vi "WMP_ess_CCL.vi"() -> ()   [LabVIEW 2013]
panel:
  out "status":string="就緒"
  out "index":i32
  out "appended path":path=path "C:/Users/TPSOP/Desktop/新增資料夾 (2)/musics/1.mp3"
  in  "Pause Button":bool
  in  "Vol.":i32(slide)=12 min=0 max=100 step=1 scale=0.0..100.0
  in  "Skip Back Button":bool
  in  "Skip Forward Button":bool
  in  "Play Button":bool
  in  "stop":bool
  in  "WindowsMediaPlayer":refnum<k7>(container)
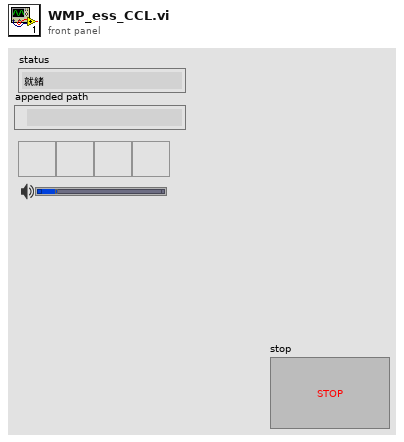
[diagram p1: front panel]
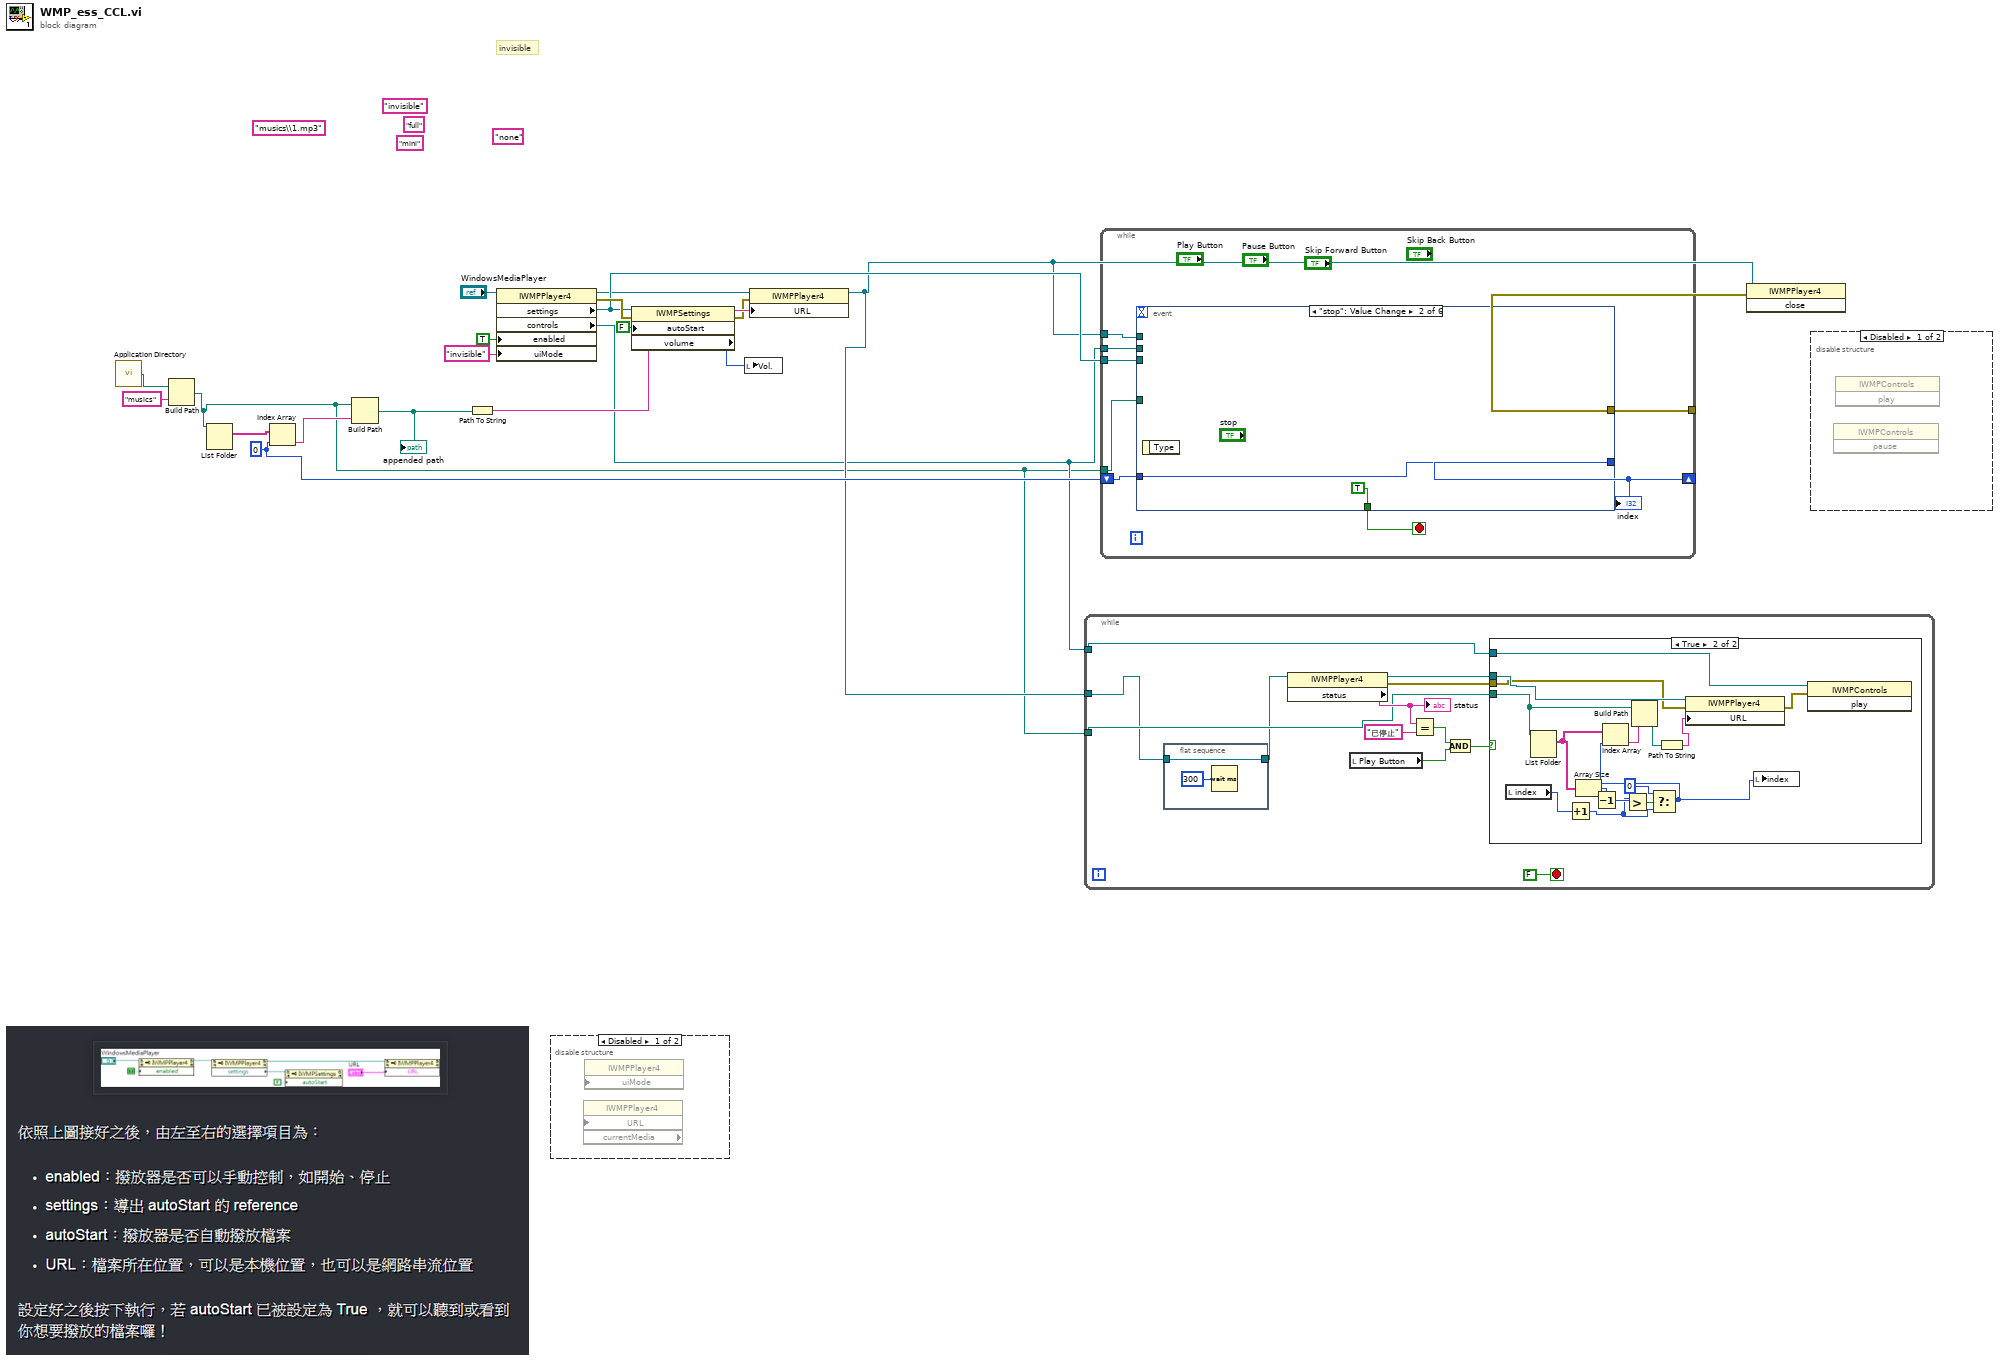
[diagram p0: block diagram]
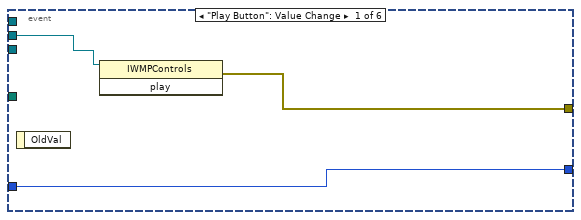
[diagram p5: hidden frame]
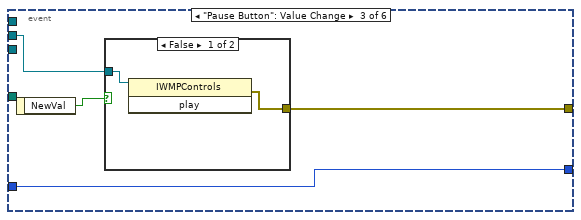
[diagram p6: hidden frame]
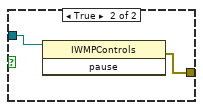
[diagram p7: hidden frame]
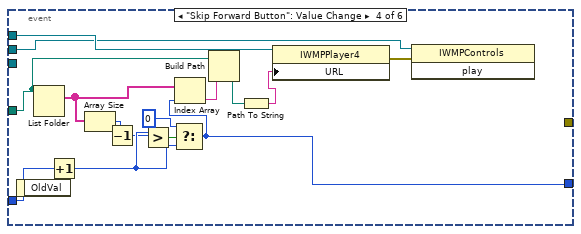
[diagram p8: hidden frame]
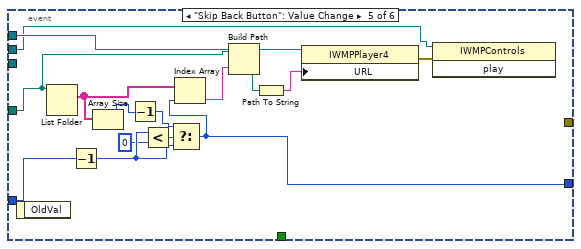
[diagram p9: hidden frame]
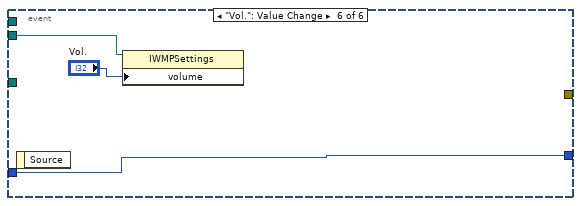
[diagram p10: hidden frame]
diagram:
  (unwired) "invisible" ("uiMode")
  (unwired) "none" ("uiMode")
  (unwired) "mini" ("uiMode")
  (unwired) "full" ("uiMode")
  w5 = 0 ("index")
  (unwired) "musics\\1.mp3" ("name or relative path")
  # "invisible"
  n1 = call <vilib>:"Application Directory.vi"() -> ("Application Directory"=w14:path)
  n2 = Build Path(base path=w14, name or relative path="musics") -> (appended path=w2:path)
  n3 = List Folder(path=w2) -> (filenames=w6:string[])  [unwired: 3 in, 3 out]
  n4 = Index Array(array=w6, index=w5) -> (element=w7:string)
  n5 = Build Path(base path=w2, name or relative path=w7) -> (appended path=w8:path)
  "appended path" <- w8
  n6 = Path To String(path=w8) -> (string=w20:string)
  n7 = property class="IWMPPlayer4"(reference="WindowsMediaPlayer", "enabled"=TRUE, "uiMode"="invisible") -> (reference out=w9:refnum<k7>, error out=w16:errorcluster, "settings"=w12:refnum<k7>, "controls"=w3:refnum<k7>)  [unwired: 1 in]
  n8 = disable-structure shown="Disabled" {
    frame Disabled {
      n9 = property class="IWMPPlayer4" props=["URL", "currentMedia"]() -> ()  [unwired: 3 in, 3 out]
      n10 = property class="IWMPPlayer4" props=["uiMode"]() -> ()  [unwired: 3 in, 2 out]
    }
    frame Enabled {
    }
  }
  n11 = property class="IWMPSettings"(reference=w12, error in=w16, "autoStart"=FALSE) -> (error out=w18:errorcluster, "volume"=w11:i32)  [unwired: 1 out]
  n12 = local write "Vol."(w11) -> ()
  n13 = property class="IWMPPlayer4"(reference=w9, error in=w18, "URL"=w20) -> (reference out=w4:refnum<k7>)  [unwired: 1 out]
  n14 = while {
    tunnel: w4 -> [w22]
    tunnel: w3 -> [w27]
    tunnel: w2 -> [w24]
    stop <- FALSE stop-if-true
    n15 = flat-sequence {
      tunnel: w22 -> [w33]
      tunnel: [w33] -> w21
      frame #0 {
        n16 = Wait (ms)(milliseconds to wait=u32 300 ("millisecond multiple")) -> ()  [unwired: 1 out]
      }
    }
    n17 = property class="IWMPPlayer4"(reference=w21) -> (reference out=w25:refnum<k7>, error out=w23:errorcluster, "status"=w31:string)  [unwired: 1 in]
    "status" <- w31
    n18 = local read "Play Button"() -> (w28:bool)
    n19 = Equal?(x=w31, y="已停止") -> (x = y?=w29:bool)
    n20 = And(x=w29, y=w28) -> (x .and. y?=w26:bool)
    n21 = case shown="True" w26 {
      tunnel: w27 -> [_ w50]
      tunnel: w25 -> [_ w39]
      tunnel: w24 -> [_ w38]
      tunnel: w23 -> [_ w35]
      frame False {
      }
      frame True {
        n22 = local read "index"() -> (w41:i32)
        n23 = List Folder(path=w38) -> (filenames=w42:string[])  [unwired: 3 in, 3 out]
        n24 = Increment(x=w41) -> (x+1=w40:i32)
        n25 = Array Size(array=w42) -> (size(s)=w48:i32)
        n26 = Decrement(x=w48) -> (x-1=w49:i32)
        n27 = Greater?(x=w40, y=w49) -> (0:w43:bool)
        n28 = Select(t=0, s=w43, f=w40) -> (s? t:f=w36:i32)
        n29 = Index Array(array=w42, index=w36) -> (element=w45:string)
        n30 = Build Path(base path=w38, name or relative path=w45) -> (appended path=w46:path)
        n31 = Path To String(path=w46) -> (string=w47:string)
        n32 = property class="IWMPPlayer4"(reference=w39, error in=w35, "URL"=w47) -> (error out=w37:errorcluster)  [unwired: 1 out]
        n33 = local write "index"(w36) -> ()
        n34 = invoke class="IWMPControls" method="play"(reference=w50, error in=w37) -> ()  [unwired: 1 in, 3 out]
      }
    }
  }
  n35 = while {
    tunnel: w3 -> [w58]
    tunnel: [w57] -> w17
    tunnel: w12 -> [w55]
    shift-right: [w51] -> _
    shift-left: w5 -> [w54]
    tunnel: w2 -> [w53]
    tunnel: w4 -> [w52]
    stop <- w56 stop-if-true
    n36 = event shown="[1] \"stop\": Value Change" {
      selector: _ -> [_ _ _ _ _ _]
      dyn-events: _ -> [_ _ _ _ _ _]
      timeout: _ -> [_ _ _ _ _ _]
      tunnel: w58 -> [w61 _ w66 w73 w87 _]
      tunnel: [w60 _ w65 _ _ _] -> w57
      tunnel: [_ TRUE _ _ _ _] -> w56
      tunnel: w55 -> [_ _ _ _ _ w103]
      tunnel: w54 -> [w59 w62 w64 w85 w100 w102]
      tunnel: w53 -> [_ _ _ w79 w93 _]
      tunnel: w52 -> [_ _ _ w86 w101 _]
      tunnel: [w59 w62 w64 w80 w95 w102] -> w51
      event "Play Button": Value Change {
        n37 = event-data() -> ()  [unwired: 1 in, 1 out]
        n38 = invoke class="IWMPControls" method="play"(reference=w61) -> (error out=w60:errorcluster)  [unwired: 2 in, 2 out]
      }
      event "stop": Value Change {
        n39 = event-data() -> ()  [unwired: 1 in, 1 out]
      }
      event "Pause Button": Value Change {
        n40 = event-data() -> ("NewVal"=w67:bool)  [unwired: 1 in]
        n41 = case shown="False" w67 {
          tunnel: w66 -> [w68 w71]
          tunnel: [w69 w70] -> w65
          frame False {
            n42 = invoke class="IWMPControls" method="play"(reference=w68) -> (error out=w69:errorcluster)  [unwired: 2 in, 2 out]
          }
          frame True {
            n43 = invoke class="IWMPControls" method="pause"(reference=w71) -> (error out=w70:errorcluster)  [unwired: 2 in, 2 out]
          }
        }
      }
      event "Skip Forward Button": Value Change {
        n44 = event-data() -> ()  [unwired: 1 in, 1 out]
        n45 = List Folder(path=w79) -> (filenames=w84:string[])  [unwired: 3 in, 3 out]
        n46 = Increment(x=w85) -> (x+1=w82:i32)
        n47 = Array Size(array=w84) -> (size(s)=w75:i32)
        n48 = Decrement(x=w75) -> (x-1=w74:i32)
        n49 = Greater?(x=w82, y=w74) -> (0:w83:bool)
        n50 = Select(t=0, s=w83, f=w82) -> (s? t:f=w80:i32)
        n51 = Index Array(array=w84, index=w80) -> (element=w78:string)
        n52 = Build Path(base path=w79, name or relative path=w78) -> (appended path=w77:path)
        n53 = Path To String(path=w77) -> (string=w76:string)
        n54 = property class="IWMPPlayer4"(reference=w86, "URL"=w76) -> (error out=w72:errorcluster)  [unwired: 1 in, 1 out]
        n55 = invoke class="IWMPControls" method="play"(reference=w73, error in=w72) -> ()  [unwired: 1 in, 3 out]
      }
      event "Skip Back Button": Value Change {
        n56 = event-data() -> ()  [unwired: 1 in, 1 out]
        n57 = List Folder(path=w93) -> (filenames=w99:string[])  [unwired: 3 in, 3 out]
        n58 = Decrement(x=w100) -> (x-1=w97:i32)
        n59 = Array Size(array=w99) -> (size(s)=w90:i32)
        n60 = Decrement(x=w90) -> (x-1=w89:i32)
        n61 = Less?(x=w97, y=0) -> (x < y?=w98:bool)
        n62 = Select(t=w89, s=w98, f=w97) -> (s? t:f=w95:i32)
        n63 = Index Array(array=w99, index=w95) -> (element=w91:string)
        n64 = Build Path(base path=w93, name or relative path=w91) -> (appended path=w94:path)
        n65 = Path To String(path=w94) -> (string=w92:string)
        n66 = property class="IWMPPlayer4"(reference=w101, "URL"=w92) -> (error out=w88:errorcluster)  [unwired: 1 in, 1 out]
        n67 = invoke class="IWMPControls" method="play"(reference=w87, error in=w88) -> ()  [unwired: 1 in, 3 out]
      }
      event "Vol.": Value Change {
        n68 = event-data() -> ()  [unwired: 1 in, 1 out]
        n69 = property class="IWMPSettings"(reference=w103, "volume"="Vol.") -> ()  [unwired: 1 in, 2 out]
      }
    }
    "index" <- w51
  }
  n70 = invoke class="IWMPPlayer4" method="close"(reference=w4, error in=w17) -> ()  [unwired: 1 in, 3 out]
  n71 = disable-structure shown="Disabled" {
    frame Disabled {
      n72 = invoke class="IWMPControls" method="pause"() -> ()  [unwired: 3 in, 3 out]
      n73 = invoke class="IWMPControls" method="play"() -> ()  [unwired: 3 in, 3 out]
    }
    frame Enabled {
    }
  }
